vi "DelayGetInfo.vi"() -> (0 "Delay position (ps)":dbl format="%#_30g", 1 "Conversion":dbl format="%#_30g")   [LabVIEW 2013]
uses:
  <vilib>/Utility/file.llb/Read From Spreadsheet File (DBL).vi
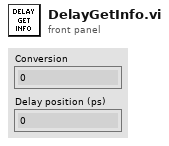
[diagram p1: front panel]
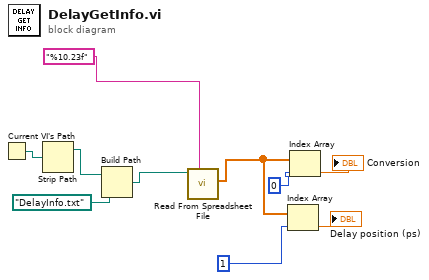
[diagram p0: block diagram]
diagram:
  n1 = Current VI's Path() -> (path=w9:path)
  n2 = Strip Path(path=w9) -> (stripped path=w8:path)  [unwired: 1 out]
  n3 = Build Path(base path=w8, name or relative path=path "DelayInfo.txt") -> (appended path=w1:path)
  n4 = call-poly <vilib>:"Read From Spreadsheet File.vi"("format (%.3f)"="%10.23f", "file path (dialog if empty)"=w1) -> ("first row"=w6:dbl[])  [unwired: 5 in, 4 out]
  n5 = Index Array(array=w6, index=1) -> (element=→"Delay position (ps)":dbl)
  n6 = Index Array(array=w6, index=0) -> (element=→"Conversion":dbl)
